vi "Get Current Dye.vi"(8 "error in (no error)":errorcluster, 11 "Settings in":refnum<class "Settings.lvclass">) -> (0 "error out":errorcluster, 1 "Selected Dye":i32, 2 "Dye Settings":T1={"Dye Name"="", "Pulse Sequence"=[], "Emission Filter"=0, "Exposure (s)"=0.01, "Yellow Select"=FALSE, "# Pulses"=0} {"Exposure (s)" min=1.0 max=5000.0}, 3 "Settings out":refnum<class "Settings.lvclass">)   [LabVIEW 2010, in "Settings.lvclass"]
uses:
  Settings.lvclass
  Settings.lvclass/Settings.ctl
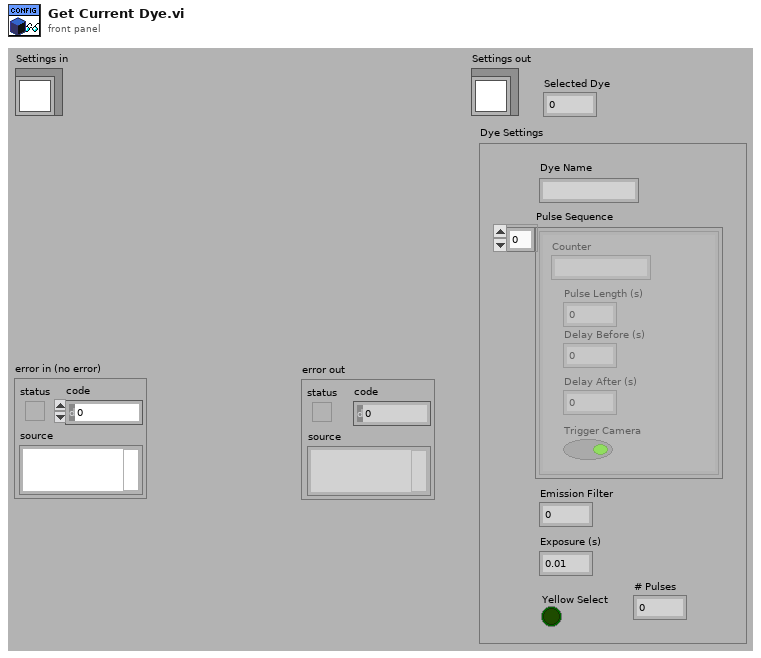
[diagram p1: front panel]
types:
  T1 = cluster{"Dye Name":string, "Pulse Sequence":cluster{"Counter":string, "Pulse Length (s)":dbl, "Delay Before (s)":dbl, "Delay After (s)":dbl, "Trigger Camera":bool}[], "Emission Filter":i16, "Exposure (s)":dbl, "Yellow Select":bool, "# Pulses":i32}
  T2 = cluster{"Dye Name":string, "Pulse Sequence":cluster{"LED Name":string, "Pulse Length (s)":dbl, "Delay Before (s)":dbl, "Delay After (s)":dbl, "Trigger Camera":bool}[], "Emission Filter":i16, "Exposure (s)":dbl, "Yellow Select":bool, "# Pulses":i32}
  T3 = cluster{"Color":string, "DLL LED Num":i32, "Wavelength":i32, "Counter Name":string, "GRN_YEL":i32, "Yellow Select":i32, "Yellow Select Line":string}[]
  T4 = cluster{"Dye Name":string, "Pulse Sequence":cluster{"LED Name":string, "Pulse Length (s)":dbl, "Delay Before (s)":dbl, "Delay After (s)":dbl, "Trigger Camera":bool}[], "Emission Filter":i16, "Exposure (s)":dbl, "Yellow Select":bool, "# Pulses":i32}[]
  T5 = cluster{"LED Name":string, "Pulse Length (s)":dbl, "Delay Before (s)":dbl, "Delay After (s)":dbl, "Trigger Camera":bool}[]
  T6 = cluster{"Counter":string, "Pulse Length (s)":dbl, "Delay Before (s)":dbl, "Delay After (s)":dbl, "Trigger Camera":bool}
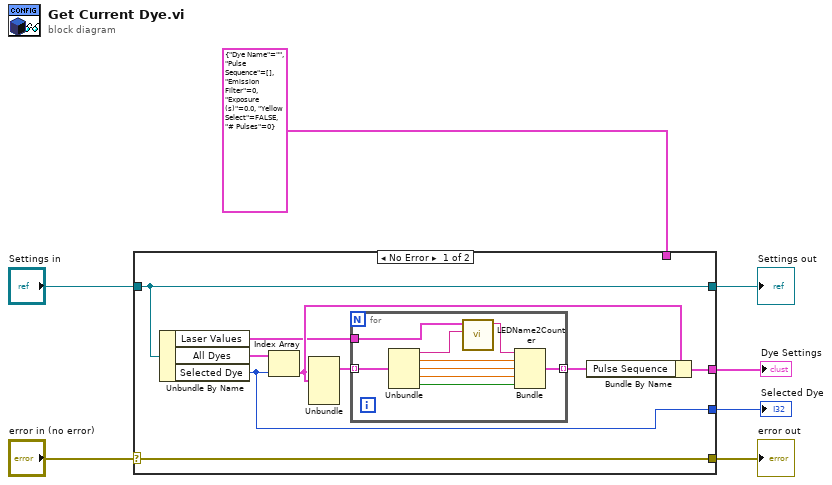
[diagram p0: block diagram]
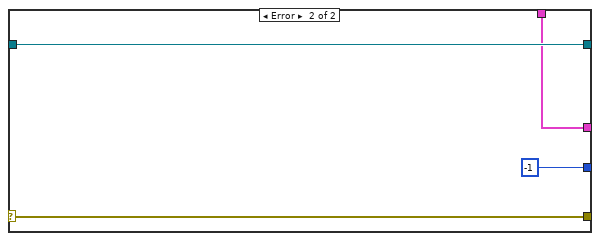
[diagram p2: hidden frame]
diagram:
  n1 = case shown="No Error" "error in (no error)" {
    selector: "error in (no error)" -> [w16 w28]
    tunnel: [w16 w28] -> w6
    tunnel: [w15 w29] -> w4
    tunnel: "Settings in" -> [w15 w29]
    tunnel: [w10 w26] -> w3
    tunnel: [w13 -1 ("Selected Dye")] -> w2
    tunnel: T2 {"Dye Name"="", "Pulse Sequence"=[], "Emission Filter"=0, "Exposure (s)"=0.0, "Yellow Select"=FALSE, "# Pulses"=0} ("Dye Settings") -> [_ w26]
    frame No Error {
      n2 = Unbundle By Name(w15) -> ("Laser Values"=w9:T3, "All Dyes"=w14:T4, "Selected Dye"=w13:i32)
      n3 = Index Array(array=w14, index=w13) -> (element=w11:T2)
      n4 = Unbundle(w11) -> ("Pulse Sequence"=w12:T5)  [unwired: 5 out]
      n5 = for {
        tunnel: w12 -> [w25] mode=indexing
        tunnel: w9 -> [w24]
        tunnel: [w17] -> w8 mode=indexing
        n6 = Unbundle(w25) -> ("LED Name"=w23:string, "Pulse Length (s)"=w21:dbl, "Delay Before (s)"=w20:dbl, "Delay After (s)"=w19:dbl, "Trigger Camera"=w18:bool)
        n7 = call "LEDName2Counter.vi"("LED Name"=w23, "LED Values"=w24) -> ("Counter"=w22:string)  [unwired: 9 in]
        n8 = Bundle("Counter"=w22, "Pulse Length (s)"=w21, "Delay Before (s)"=w20, "Delay After (s)"=w19, "Trigger Camera"=w18) -> (w17:T6)  [unwired: 1 in]
      }
      n9 = Bundle By Name(cluster=w11, "Pulse Sequence"=w8) -> (w10:T2)
    }
    frame Error {
    }
  }
  "error out" <- w6
  "Settings out" <- w4
  "Dye Settings" <- w3
  "Selected Dye" <- w2
